vi "CheckWashIndicators.vi"() -> ()   [LabVIEW 2019]
uses:
  Controls/Car Wash Indicators.ctl
panel:
  out "Car Wash OUT":T1
  in  "Car Wash IN":T1
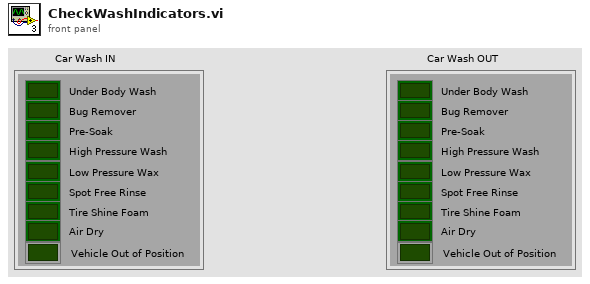
[diagram p1: front panel]
types:
  T1 = typedef "Car Wash Indicators.ctl" = cluster{"Under Body Wash":bool, "Bug Remover":bool, "Pre-Soak":bool, "High Pressure Wash":bool, "Low Pressure Wax":bool, "Spot Free Rinse":bool, "Tire Shine Foam":bool, "Air Dry":bool, "Vehicle Out of Position":bool}
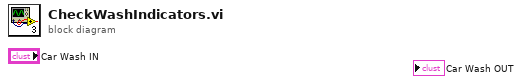
[diagram p0: block diagram]
diagram:
